vi "WriteBinaryWaveformFile.vi"(2 "Time base":dbl format="%.2e", 3 "Delay, points":dbl format="%.2f", 6 "append to file? (new file:F)":bool, 7 "Interactive":bool=TRUE, 8 "error in (no error)":errorcluster, 9 "1D array":sgl[](array[numeric]) format="%.2f", 10 "2D array":sgl[][](array[numeric]) format="%.3f", 11 "file path (dialog if empty)":path) -> (0 "error out":errorcluster, 5 "new file path (Not A Path if cancelled)":path)   [LabVIEW 2015]
doc: "Writes a 2D or 1D array of single-precision numbers (SGL) to a new byte stream file or appends the data to an existing file. The VI opens or creates the file beforehand and closes it afterwards. You can use this VI to write scaled data from data acquisition VIs.\n\nfile path is the path name of the file. If file path is empty (default value) or is Not A Path, the VI displays a File dialog box from which you can select a file. Error 43 occurs if the user cancels the dialog. \n\n2D data contains the single-precision numbers the VI writes to the file if 1D data is not wired or empty.\n\n1D data contains the single-precision numbers the VI writes to the file if this input is not empty.\n\nappend to file? Set to TRUE if you want to append the data to a existing file; you can also set it TRUE to write to a new file. Set to FALSE (default value) if you want to write the data to a new file or to replace an existing file.\n\nnew file path is the path of the file to which the VI wrote data. You can use this output to determine the path of a file that you open using dialog. new file path returns Not A Path if the user selects Cancel from the dialog box."
panel:
  in  "prompt":string="Choose file to write."
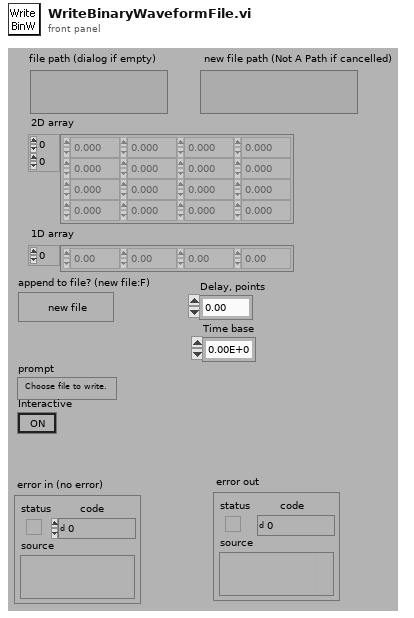
[diagram p1: front panel]
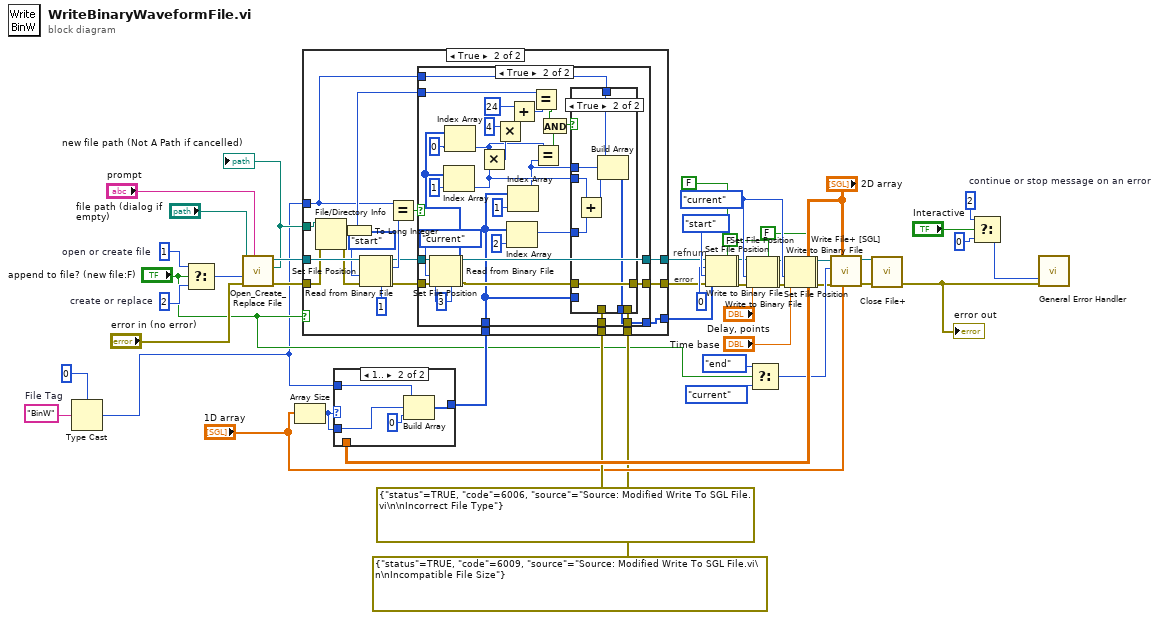
[diagram p0: block diagram]
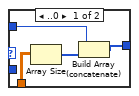
[diagram p5: hidden frame]
diagram:
  w18 = enum16{"start", "end", "current"}."current" ("pos mode (0:2)")
  w20 = "BinW"  # File Tag
  w47 = i16 2  # create or replace
  w44 = 2  # continue or stop message on an error
  w48 = i16 1  # open or create file
  # "error"
  # "refnum"
  n1 = Type Cast(type=0, x=w20) -> (*(type *) &x=w19:i32)
  n2 = Select(t=w48, s="append to file? (new file:F)", f=w47) -> (s? t:f=w49:i16)
  n3 = call <vilib>:"Open_Create_Replace File.vi"("prompt"="prompt", "error in (no error)"="error in (no error)", "function (open:0)"=w49, "file path"="file path (dialog if empty)") -> ("error out"=w36:errorcluster, "new file path"=w31:path, "refnum"=w35:refnum<file>)  [unwired: 2 in, 3 out]
  "new file path (Not A Path if cancelled)" <- w31
  n4 = Array Size(array="1D array") -> (size(s)=w27:i32)
  n5 = case shown="1.." w27 {
    tunnel: "2D array" -> [w56 _]
    tunnel: [w54 w60] -> w30
    tunnel: w19 -> [w53 w57]
    tunnel: w27 -> [_ w58]
    frame ..0 {
      n6 = Array Size(array=w56) -> (size(s)=w55:i32[])
      n7 = Build Array (concatenate)(w53, w55) -> (w54:i32[])
    }
    frame 1.. {
      n8 = Build Array(w57, w58, 0 ("Input Element")) -> (w60:i32[])
    }
  }
  n9 = case shown="True" "append to file? (new file:F)" {
    tunnel: w36 -> [w62 w73]
    tunnel: w35 -> [w63 w84]
    tunnel: w19 -> [_ w68]
    tunnel: [w62 w79] -> w34
    tunnel: errorcluster {"status"=TRUE, "code"=6006, "source"="Source: Modified Write To SGL File.vi\n\nIncorrect File Type"} ("error out") -> [_ w78]
    tunnel: [w63 w77] -> w32
    tunnel: w31 -> [_ w74]
    tunnel: w30 -> [w61 w70]
    tunnel: [w61 w69] -> w29
    tunnel: errorcluster {"status"=TRUE, "code"=6009, "source"="Source: Modified Write To SGL File.vi\n\nIncompatible File Size"} ("error out") -> [_ w67]
    frame False {
    }
    frame True {
      n10 = File/Directory Info(path=w74, error in=w73) -> (size=w66:i64, error out=w72:errorcluster)  [unwired: 5 out]
      n11 = To Long Integer(number=w66) -> (32bit integer=w71:i32)
      n12 = Set File Position(refnum=w84, from (0:start)=enum16{"start", "end", "current"}."start" ("pos mode (0:2)"), error in=w72) -> (refnum out=w65:refnum<file>, error out=w64:errorcluster)  [unwired: 1 out]
      n13 = Read from Binary File(5:1 ("count"), 8:w64, 11:w65) -> (0:w75:errorcluster, 2:w82:i32, 3:w76:refnum<file>)  [unwired: 4 out]
      n14 = Equal?(x=w68, y=w82) -> (x = y?=w80:bool)
      n15 = case shown="True" w80 {
        tunnel: [w87 w100] -> w79
        tunnel: w78 -> [w87 w99]
        tunnel: [w86 w98] -> w77
        tunnel: w76 -> [w86 w118]
        tunnel: w75 -> [_ w115]
        tunnel: w71 -> [_ w108]
        tunnel: w70 -> [w85 w91]
        tunnel: [w85 w92] -> w69
        tunnel: w68 -> [_ w94]
        tunnel: w67 -> [_ w90]
        frame False {
        }
        frame True {
          w116 = 3 ("count")
          n16 = Set File Position(refnum=w118, from (0:start)=enum16{"start", "end", "current"}."current" ("pos mode (0:2)"), error in=w115) -> (refnum out=w89:refnum<file>, error out=w88:errorcluster)  [unwired: 1 out]
          n17 = Read from Binary File(5:w116, 8:w88, 10:w116, 11:w89) -> (0:w101:errorcluster, 2:w119:i32[], 3:w98:refnum<file>)  [unwired: 3 out]
          n18 = Index Array(array=w119, index=1 ("Index")) -> (element=w97:i32)
          n19 = Index Array(array=w119, index=0 ("Index")) -> (element=w106:i32)
          n20 = Multiply(x=w106, y=w97) -> (x*y=w112:i32)
          n21 = Multiply(x=4, y=w112) -> (x*y=w110:i32)
          n22 = Index Array(array=w91, index=2 ("Index")) -> (element=w95:i32)
          n23 = Index Array(array=w91, index=1 ("Index")) -> (element=w93:i32)
          n24 = Add(x=24, y=w110) -> (x+y=w107:i32)
          n25 = Equal?(x=w108, y=w107) -> (x = y?=w104:bool)
          n26 = Equal?(x=w106, y=w93) -> (x = y?=w103:bool)
          n27 = And(x=w104, y=w103) -> (x .and. y?=w102:bool)
          n28 = case shown="True" w102 {
            tunnel: w101 -> [_ w128]
            tunnel: [w120 w128] -> w100
            tunnel: w99 -> [_ _]
            tunnel: w97 -> [_ w127]
            tunnel: w95 -> [_ w126]
            tunnel: w94 -> [_ w122]
            tunnel: w93 -> [_ w124]
            tunnel: [w121 w123] -> w92
            tunnel: w91 -> [w121 _]
            tunnel: w90 -> [w120 _]
            frame False {
            }
            frame True {
              n29 = Add(x=w127, y=w126) -> (x+y=w125:i32)
              n30 = Build Array(w122, w124, w125) -> (w123:i32[])
            }
          }
        }
      }
    }
  }
  n31 = Set File Position(offset (in bytes) (0)=0 ("pos offset (0)"), refnum=w32, from (0:start)=enum16{"start", "end", "current"}."start" ("pos mode (0:2)"), error in=w34) -> (refnum out=w3:refnum<file>, error out=w2:errorcluster)
  n32 = Write to Binary File(file (use dialog)=w3, data=w29, error in=w2, 5:FALSE ("prepend array or string size? (T)")) -> (refnum out=w17:refnum<file>, error out=w14:errorcluster)  [unwired: 3 out]
  n33 = Set File Position(refnum=w17, from (0:start)=w18, error in=w14) -> (refnum out=w6:refnum<file>, error out=w5:errorcluster)  [unwired: 1 out]
  n34 = Write to Binary File(file (use dialog)=w6, data="Delay, points", error in=w5, 5:FALSE ("prepend array or string size? (T)")) -> (refnum out=w16:refnum<file>, error out=w15:errorcluster)  [unwired: 3 out]
  n35 = Select(t=enum16{"start", "end", "current"}."end" ("pos mode (rel. to end:1)"), s="append to file? (new file:F)", f=enum16{"start", "end", "current"}."current" ("pos mode (rel. to end:1)")) -> (s? t:f=w22:enum16{"start", "end", "current"})
  n36 = Set File Position(refnum=w16, from (0:start)=w18, error in=w15) -> (refnum out=w9:refnum<file>, error out=w8:errorcluster)  [unwired: 1 out]
  n37 = Write to Binary File(file (use dialog)=w9, data="Time base", error in=w8, 5:FALSE ("prepend array or string size? (T)")) -> (refnum out=w12:refnum<file>, error out=w13:errorcluster)  [unwired: 3 out]
  n38 = call <vilib>:"Write File+ [SGL].vi"("1D array"="1D array", "2D array"="2D array", "error in (no error)"=w13, "pos mode (rel. to end:1)"=w22, "refnum"=w12) -> ("error out"=w51:errorcluster, "dup refnum"=w50:refnum<file>)  [unwired: 1 in, 4 out]
  n39 = call <vilib>:"Close File+.vi"("error in (no error)"=w51, "refnum"=w50) -> ("error out"=w37:errorcluster)  [unwired: 5 out]
  "error out" <- w37
  n40 = Select(t=w44, s="Interactive", f=0) -> (s? t:f=w42:i32)
  n41 = call <vilib>:"General Error Handler.vi"("type of dialog (OK msg:1)"=w42, "error in (no error)"=w37) -> ()  [unwired: 1 in, 13 out]
